vi "TtoV.vi"(1 "Temp":dbl) -> (0 "Volt":dbl)   [LabVIEW 2016]
doc: "Подпрограмма предназначена для перевода температуры\nв диапазоне 0-40 оС в напряжение 0-5В для дальнейшей\nвыдачи сигнала на DAQ"
panel:
  # "Подпрограмма предназначена для перевода температуры\nв диапазоне 0-40 оС в напряжение 0-5В для дальнейшей\nвыдачи сигнала на DAQ"
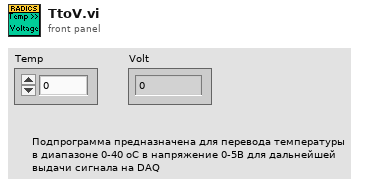
[diagram p1: front panel]
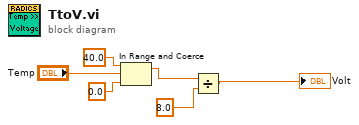
[diagram p0: block diagram]
diagram:
  n1 = In Range and Coerce(upper limit=40.0, x="Temp", lower limit=0.0) -> (coerced(x)=w1:dbl)  [unwired: 1 out]
  n2 = Divide(x=w1, y=8.0) -> (x/y=→"Volt":dbl)
